vi "Check Max Cycles.vi"(8 "error in (no error)":errorcluster, 11 "Output Sequencer in":refnum<class "Output Sequencer.lvclass">) -> (0 "error out":errorcluster, 2 "Max iterations reached?":bool, 3 "Output Sequencer out":refnum<class "Output Sequencer.lvclass">, 5 "Sequencer State":T1)   [LabVIEW 2020, in "Output Sequencer.lvlib" / "Output Sequencer.lvclass"]
uses:
  Output Sequencer.lvclass
  Types/Sequencer State.ctl
  Output Sequencer.lvclass/Output Sequencer.ctl
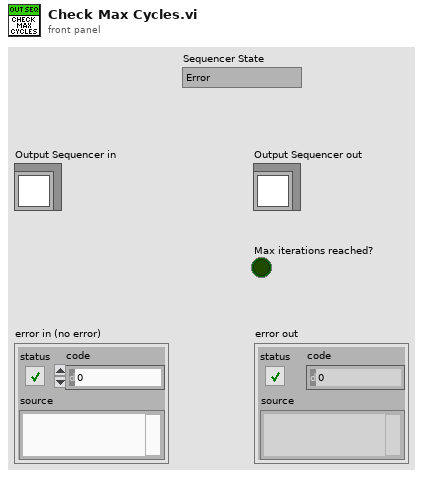
[diagram p1: front panel]
types:
  T1 = typedef "Output Sequencer.lvlib/Output Sequencer.lvclass/Sequencer State.ctl" = enum16{"Error", "Initialize", "Prepare channels", "Wait for test", "Wait for %.1f sec", "Wait for trigger", "Stop condition", "Wait for resume", "Running", "Paused", "Stopped"}
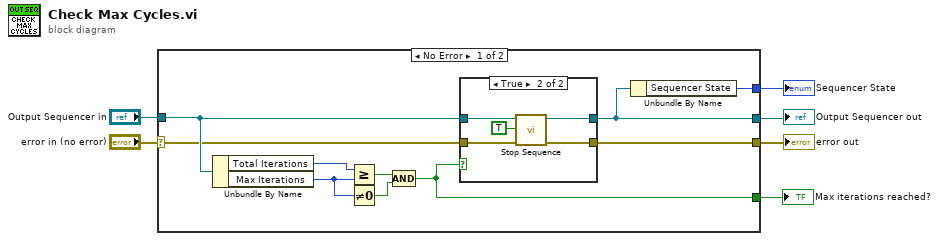
[diagram p0: block diagram]
diagram:
  n1 = case shown="No Error" "error in (no error)" {
    selector: "error in (no error)" -> [w7 w25]
    tunnel: [w12 _] -> w6
    tunnel: "Output Sequencer in" -> [w11 w24]
    tunnel: [w10 w25] -> w4
    tunnel: [w9 w24] -> w3
    tunnel: [w8 _] -> w2
    frame No Error {
      n2 = Unbundle By Name(w11) -> ("Total Iterations"=w16:i32, "Max Iterations"=w15:u32)
      n3 = Greater Or Equal?(x=w16, y=w15) -> (x >= y?=w14:bool)
      n4 = Not Equal To 0?(x=w15) -> (x != 0?=w13:bool)
      n5 = Compound Arithmetic op=AND(w14, w13) -> (w12:bool)
      n6 = case shown="True" w12 {
        tunnel: w11 -> [w18 w23]
        tunnel: [w18 w22] -> w9
        tunnel: w7 -> [w17 w20]
        tunnel: [w17 w19] -> w10
        frame False {
        }
        frame True {
          n7 = call "Stop Sequence.vi"("error in (no error)"=w20, "Use previous step values for Last values"=TRUE, "Output Sequencer in"=w23) -> ("error out"=w19:errorcluster, "Output Sequencer out"=w22:refnum<class "Output Sequencer.lvclass">)  [unwired: 6 in, 1 out]
        }
      }
      n8 = Unbundle By Name(w9) -> ("Sequencer State"=w8:T1)
    }
    frame Error {
    }
  }
  "Output Sequencer out" <- w3
  "Max iterations reached?" <- w6
  "error out" <- w4
  "Sequencer State" <- w2
